vi "Find Public API VIs.vi"(8 "error in":errorcluster, 11 "Library in":refnum<vi>) -> (0 "error out":errorcluster, 3 "Public API VIs Paths":path[](array[path]))   [LabVIEW 2020, in "Panther Dashboard.lvlib" / "Library.lvclass"]
uses:
  Library.lvclass
  Panther Dashboard/Public VIs names--enum.ctl
  Panther Dashboard/Panther Dashboard.lvlib
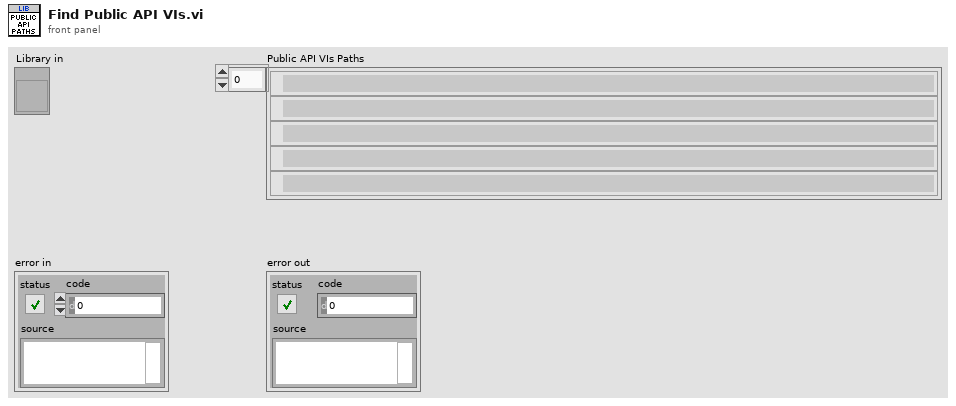
[diagram p1: front panel]
types:
  T1 = typedef "Panther Dashboard.lvlib/Public VIs names--enum.ctl" = enum16{"Start Module.vi", "Synchronize Module Events.vi", "Obtain Broadcast Events for Registration.vi", "Null Broadcast Events--constant.vi", "Stop Module.vi", "Load Module.vi", "Obtain Default Broadcast Events.vi"}
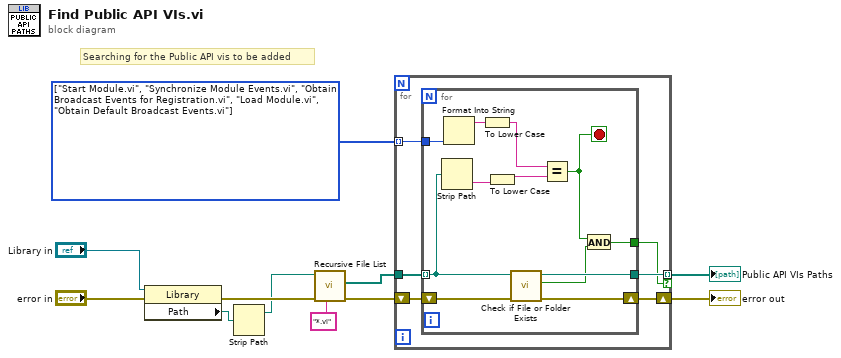
[diagram p0: block diagram]
diagram:
  w6 = T1[] [enum."Start Module.vi", enum."Synchronize Module Events.vi", enum."Obtain Broadcast Events for Registration.vi", enum."Load Module.vi", enum."Obtain Default Broadcast Events.vi"] items=["Start Module.vi", "Synchronize Module Events.vi", "Obtain Broadcast Events for Registration.vi", "Null Broadcast Events--constant.vi", "Stop Module.vi", "Load Module.vi", "Obtain Default Broadcast Events.vi"]
  # "Searching for the Public API vis to be added"
  n1 = property class="Library"(reference="Library in", error in="error in") -> (error out=w10:errorcluster, "Path"=w3:path)  [unwired: 1 out]
  n2 = Strip Path(path=w3) -> (stripped path=w2:path)  [unwired: 1 out]
  n3 = call <vilib>:"Recursive File List.vi"("pattern"="*.vi", "error in (no error)"=w10, "Folder Path"=w2) -> ("error out"=w9:errorcluster, "All Files in Dir"=w5:path[])  [unwired: 4 in, 3 out]
  n4 = for {
    tunnel: w6 -> [w15] mode=indexing
    tunnel: w5 -> [w14]
    tunnel: [w13] -> w4 mode=indexing if=w12
    shift-right: [w16] -> w8
    shift-left: w9 -> [w17]
    n5 = for {
      tunnel: w15 -> [w27]
      tunnel: w14 -> [w23] mode=indexing
      tunnel: [w25] -> w13
      shift-right: [w28] -> w16
      shift-left: w17 -> [w29]
      tunnel: [w18] -> w12
      stop <- w19 stop-if-true
      n6 = Strip Path(path=w23) -> (name=w22:string)  [unwired: 1 out]
      n7 = Format Into String(w27) -> (resulting string=w26:string)  [unwired: 3 in, 1 out]
      n8 = To Lower Case(string=w26) -> (all lower case string=w20:string)
      n9 = To Lower Case(string=w22) -> (all lower case string=w21:string)
      n10 = call <vilib>:"Check if File or Folder Exists.vi"("error in (no error)"=w29, "path"=w23) -> ("error out"=w28:errorcluster, "file or folder exists?"=w24:bool, "dup path"=w25:path)  [unwired: 7 in]
      n11 = Equal?(x=w20, y=w21) -> (x = y?=w19:bool)
      n12 = And(x=w19, y=w24) -> (x .and. y?=w18:bool)
    }
  }
  "Public API VIs Paths" <- w4
  "error out" <- w8
